vi "File_Browser.vi"(9 "FileIndexIn":i32, 10 "FileExt":string, 11 "FolderPath":path) -> (0 "Last?":bool, 1 "FileIndexOut":i32, 2 "FileTotal":i32, 3 "FullFilePath":path, 4 "First?":bool, 5 "FileName":string)   [LabVIEW 2009]
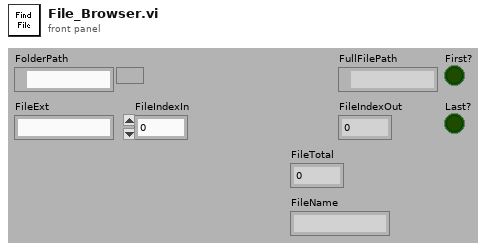
[diagram p1: front panel]
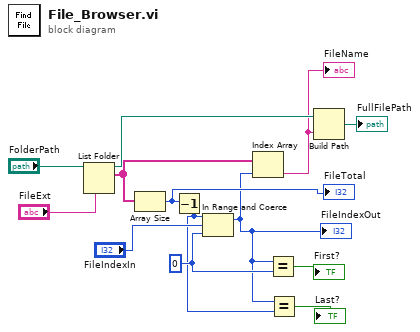
[diagram p0: block diagram]
diagram:
  w5 = 0 ("lower limit")
  n1 = List Folder(path="FolderPath", pattern="FileExt") -> (path out=w8:path, filenames=w11:string[])  [unwired: 2 in, 2 out]
  n2 = Array Size(array=w11) -> (size(s)=w10:i32)
  "FileTotal" <- w10
  n3 = Decrement(x=w10) -> (x-1=w3:i32)
  n4 = In Range and Coerce(upper limit=w3, x="FileIndexIn", lower limit=w5) -> (coerced(x)=w2:i32)  [unwired: 1 out]
  "FileIndexOut" <- w2
  n5 = Index Array(array=w11, index=w2) -> (element=w7:string)
  "FileName" <- w7
  n6 = Equal?(x=w2, y=w5) -> (x = y?=→"First?":bool)
  n7 = Equal?(x=w2, y=w3) -> (x = y?=→"Last?":bool)
  n8 = Build Path(base path=w8, name or relative path=w7) -> (appended path=→"FullFilePath":path)
